vi "Main.vi"(11 "Module Admin":refnum<class "Delacor_lib_QMH_Cloneable Module Admin.lvclass">) -> ()   [LabVIEW 2021, in "Slave.lvlib"]
doc: "This template is based off of the Queued Message Handler design pattern and the Queued Message Handler project template that ships with LabVIEW.\n\nThe main difference is that the queue is private to this module and communication between modules is performed via Broadcast and Request events.\n\nRequest events are wrapped in public API methods and are handled in the Event Handling Loop (EHL) of this VI. Any module can register for Broadcast events sent by this module. The EHL generates messages based on user interface actions.\n\nThe Message Handling Loop (MHL) processes messages generated by the EHL, or by other messages. The messages are string values, so new messages can be added easily to the Message Cases case structure in the MHL. Each message cluster can also provide an optional value for Message Data, which is a variant that can be converted to whatever message-specific data is required.\n_____\nBased on DQMH Project Template 6.1.0.94.\n\n<b>Note:</b> This VI was modified by the <b>Validate DQMH Module</b> tool to add a 'Panel Hidden' status updated broadcast to the Panel Close? event when External Launch = TRUE.\n\n<b>Note:</b> This VI was modified by the <b>Validate DQMH Module</b> tool to add a call to the Error Reported VI at the end of the 'Exit' MHL frame."
uses:
  Slave.lvlib
  <vilib>/Delacor/Delacor QMH/Libraries/Cloneable Module Admin_class/Delacor_lib_QMH_Cloneable Module Admin.lvclass
  C:/Program Files/National Instruments/LabVIEW 2021/vi.lib/Delacor/Delacor QMH/Libraries/Module Admin_class/Delacor_lib_QMH_Module Admin.lvclass
  <vilib>/Delacor/Delacor QMH/Libraries/Cloneable Module Admin_class/Delacor_lib_QMH_Cloneable Module Admin.lvclass/Delacor_lib_QMH_Cloneable Module Admin.ctl
  Module Data--cluster.ctl
  <vilib>/Delacor/Delacor QMH/Libraries/Message Queue_class/Delacor_lib_QMH_Message Queue.lvclass/Delacor_lib_QMH_Message Queue.ctl
  Stop Argument--cluster.ctl
  <vilib>/Delacor/Delacor QMH/Libraries/Module Admin_class/Delacor_lib_QMH_Module Admin.lvclass/Delacor_lib_QMH_Module Admin.ctl
  <vilib>/Utility/miscctls.llb/LVPointTypeDef.ctl
  <vilib>/Delacor/Delacor QMH/Libraries/Message Queue_class/Delacor_lib_QMH_Enqueue Message (Single).vi
  <vilib>/Delacor/Delacor QMH/Libraries/Cloneable Module Admin_class/Delacor_lib_QMH_Get Module ID.vi
  <vilib>/Delacor/Delacor QMH/Libraries/Module Admin_class/Delacor_lib_QMH_Get External Launch.vi
  <vilib>/Utility/error.llb/Error Cluster From Error Code.vi
  <vilib>/ErrorRing/Error Ring.xnode
  <vilib>/Delacor/Delacor QMH/Libraries/Message Queue_class/Delacor_lib_QMH_Message Queue.lvclass
  <vilib>/DQMH Consortium/Lumos API/Libraries/SDV API/SDV API.lvlib
panel:
  out "Title":string
  out "error out":errorcluster
  out "Status":string
  in  "Simulate EHL Error":bool
  in  "Simulate MHL Error":bool
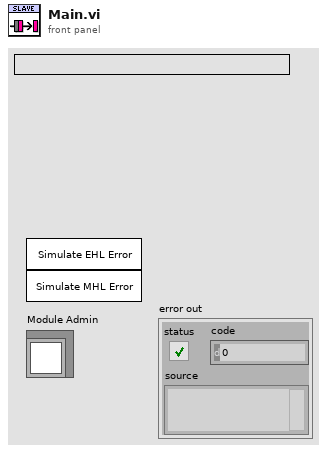
[diagram p1: front panel]
types:
  T1 = typedef "Slave.lvlib/Request Events--cluster.ctl" = cluster{"Stop Module":refnum<user-event>, "Show Panel":refnum<user-event>, "Hide Panel":refnum<user-event>, "Show Diagram":refnum<user-event>, "Get Module Execution Status":refnum<user-event>}
  T2 = typedef "Slave.lvlib/Module Data--cluster.ctl" = cluster{"Status":string}
  T3 = enum32{"invalid lock state", "Not Locked", "Locked (No Password)", "Password-protected"}
  T4 = typedef "Slave.lvlib/Stop Argument--cluster.ctl" = cluster{"Module ID":i32, "Origin":string, "Exit via Stop Module Req?":bool, "Wait for Module to stop?":bool}
  T5 = typedef "LVPointTypeDef.ctl" = cluster{"Horizontal":i16, "Vertical":i16}
  T6 = enum32{"Invalid", "Standard", "Closed", "Hidden", "Minimized", "Maximized"}
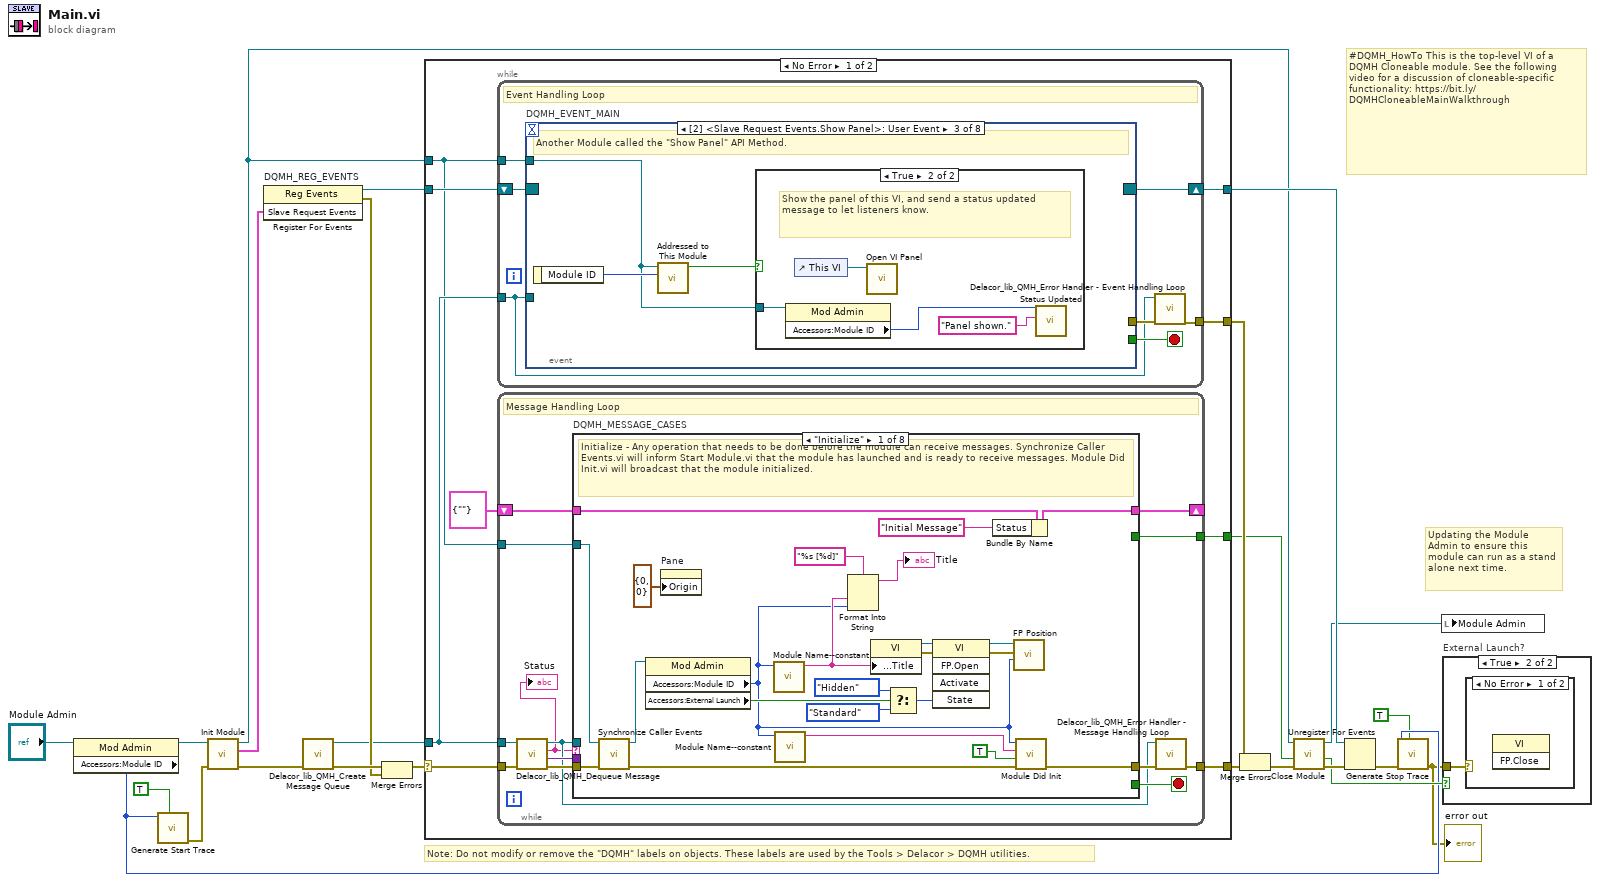
[diagram p0: block diagram]
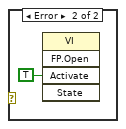
[diagram p3: hidden frame]
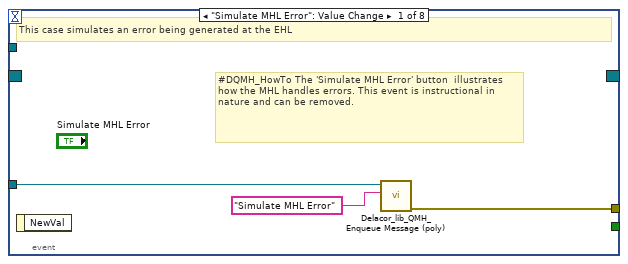
[diagram p4: hidden frame]
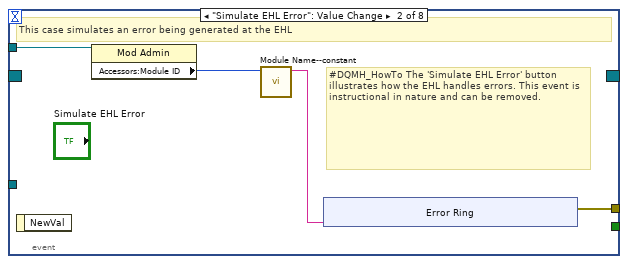
[diagram p5: hidden frame]
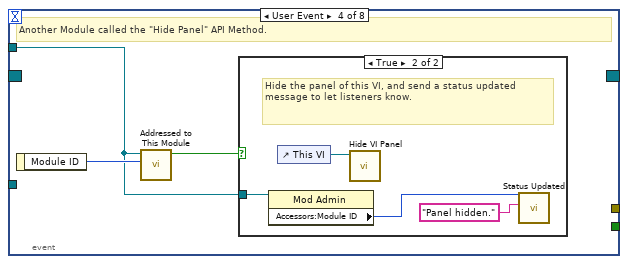
[diagram p7: hidden frame]
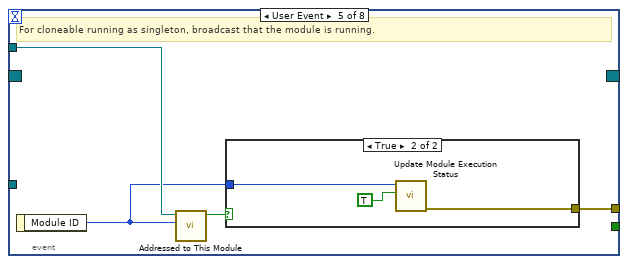
[diagram p9: hidden frame]
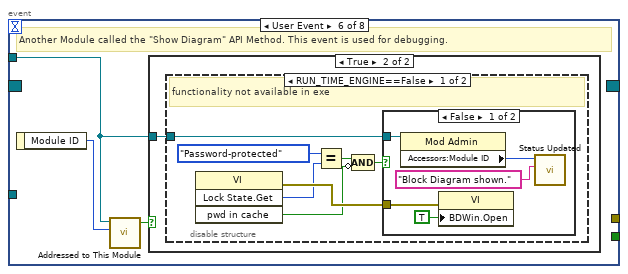
[diagram p11: hidden frame]
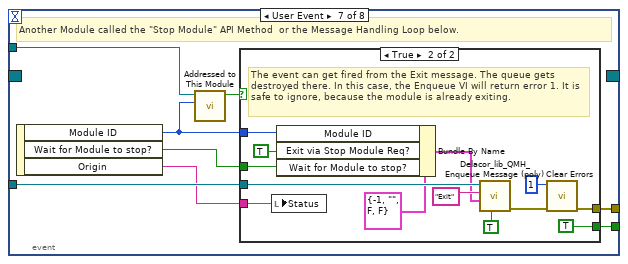
[diagram p15: hidden frame]
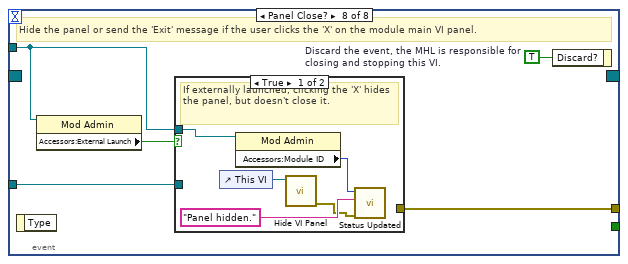
[diagram p17: hidden frame]
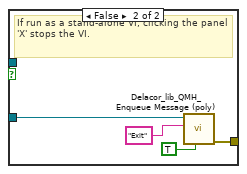
[diagram p18: hidden frame]
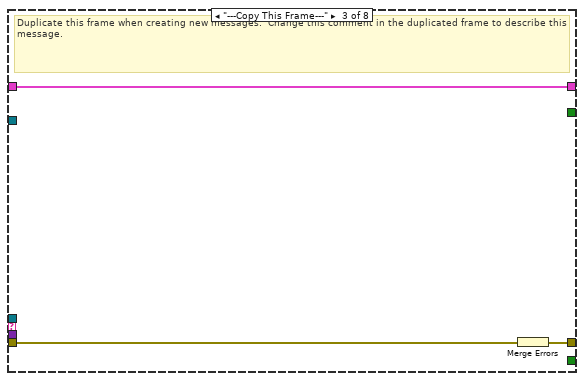
[diagram p20: hidden frame]
diagram:
  # "#DQMH_HowTo This is the top-level VI of a DQMH Cloneable module. See the following video for a discussion of cloneable-specific functionality: https://bit.ly/DQMHCloneableMainWalkthrough"
  # "Note: Do not modify or remove the \"DQMH\" labels on objects. These labels are used by the Tools > Delacor > DQMH utilities."
  # "Updating the Module Admin to ensure this module can run as a stand alone next time."
  n1 = property on="Property Node" class="Mod Admin"(reference="Module Admin") -> (reference out=w6:refnum<class "Delacor_lib_QMH_Cloneable Module Admin.lvclass">, "Accessors:Module ID"=w4:i32)  [unwired: 1 in, 1 out]
  n2 = call <vilib>:"Generate Start Trace.vi"("Reply (F)"=TRUE, "Module ID (0)"=w4) -> ("error out"=w5:errorcluster)  [unwired: 9 in]
  n3 = call "Init Module.vi"("error in"=w5, "Cloneable Module Admin in"=w6) -> ("error out"=w21:errorcluster, "Slave Request Events"=w13:T1, "Cloneable Module Admin out"=w10:refnum<class "Delacor_lib_QMH_Cloneable Module Admin.lvclass">)  [unwired: 7 in]
  n4 = register-events "DQMH_REG_EVENTS"(w13) -> (reference out=w14:refnum<event-registration>, error out=w16:errorcluster)  [unwired: 2 in]
  n5 = call <vilib>:"Delacor_lib_QMH_Create Message Queue.vi"("error in"=w21) -> ("error out"=w18:errorcluster, "Message Queue"=w12:refnum<class "Delacor_lib_QMH_Message Queue.lvclass">)  [unwired: 9 in]
  n6 = Merge Errors(w18, w16) -> (w17:errorcluster)
  n7 = case shown="No Error" w17 {
    selector: w17 -> [w31 w236]
    tunnel: [w33 w235] -> w22
    tunnel: [w30 w243] -> w15
    tunnel: w14 -> [w28 w243]
    tunnel: w12 -> [w27 w234]
    tunnel: [w32 _] -> w23
    tunnel: w10 -> [w26 w239]
    tunnel: [w25 _] -> w8
    frame No Error {
      n8 = while {
        tunnel: w27 -> [w34]
        shift-right: [w37] -> w30
        shift-left: w28 -> [w38]
        tunnel: [w39] -> w32
        tunnel: w26 -> [w35]
        stop <- w36 stop-if-true
        # "Event Handling Loop"
        n9 = event "DQMH_EVENT_MAIN" shown="[2] <Slave Request Events.Show Panel>: User Event" {
          selector: w38 -> [_ _ _ _ _ _ _ _]
          dyn-events: [_ _ _ _ _ _ _ _] -> w37
          timeout: _ -> [_ _ _ _ _ _ _ _]
          tunnel: [_ _ _ _ _ _ w95 _] -> w36
          tunnel: w34 -> [w42 _ _ _ _ _ w98 w115]
          tunnel: [w43 w47 _ _ w72 _ w99 w117] -> w40
          tunnel: w35 -> [_ w46 w55 w62 w70 w76 w97 w113]
          event "Simulate MHL Error": Value Change {
            # "#DQMH_HowTo The 'Simulate MHL Error' button  illustrates how the MHL handles errors. This event is instructional in nature and can be removed."
            # "This case simulates an error being generated at the EHL"
            n10 = event-data() -> ()  [unwired: 1 in, 1 out]
            n11 = call-poly <vilib>:"Delacor_lib_QMH_Enqueue Message (poly).vi"("Message"="Simulate MHL Error", "Message Queue in"=w42) -> ("error out"=w43:errorcluster)  [unwired: 8 in, 1 out]
          }
          event "Simulate EHL Error": Value Change {
            # "#DQMH_HowTo The 'Simulate EHL Error' button  illustrates how the EHL handles errors. This event is instructional in nature and can be removed."
            # "This case simulates an error being generated at the EHL"
            n12 = event-data() -> ()  [unwired: 1 in, 1 out]
            n13 = property on="Property Node" class="Mod Admin"(reference=w46) -> ("Accessors:Module ID"=w45:i32)  [unwired: 1 in, 2 out]
            n14 = call "Module Name--constant.vi"("Module ID"=w45) -> ("Module Name"=w44:string)  [unwired: 10 in]
            n15 = xnode ("Error Ring")("parameter 0"=w44) -> ("error out"=w47:errorcluster)
          }
          event User Event {
            # "Another Module called the \"Show Panel\" API Method."
            n16 = event-data() -> ("Module ID"=w56:i32)  [unwired: 1 in]
            n17 = call "Addressed to This Module.vi"("Module ID from Argument"=w56, "Module Admin"=w55) -> ("Addressed to this instance?"=w57:bool)  [unwired: 8 in, 1 out]
            n18 = case shown="True" w57 {
              tunnel: w55 -> [_ w59]
              frame False {
              }
              frame True {
                # "Show the panel of this VI, and send a status updated message to let listeners know."
                n19 = property on="Property Node" class="Mod Admin"(reference=w59) -> ("Accessors:Module ID"=w58:i32)  [unwired: 1 in, 2 out]
                n20 = control-ref of="This VI"() -> (w61:refnum<vi>)
                n21 = call "Open VI Panel.vi"("VI"=w61) -> ()  [unwired: 10 in, 1 out]
                n22 = call "Status Updated.vi"("Status"="Panel shown." ("format string"), "Module ID"=w58) -> ()  [unwired: 9 in, 1 out]
              }
            }
          }
          event User Event {
            # "Another Module called the \"Hide Panel\" API Method."
            n23 = event-data() -> ("Module ID"=w63:i32)  [unwired: 1 in]
            n24 = call "Addressed to This Module.vi"("Module ID from Argument"=w63, "Module Admin"=w62) -> ("Addressed to this instance?"=w64:bool)  [unwired: 8 in, 1 out]
            n25 = case shown="True" w64 {
              tunnel: w62 -> [_ w66]
              frame False {
              }
              frame True {
                # "Hide the panel of this VI, and send a status updated message to let listeners know."
                n26 = property on="Property Node" class="Mod Admin"(reference=w66) -> ("Accessors:Module ID"=w65:i32)  [unwired: 1 in, 2 out]
                n27 = control-ref of="This VI"() -> (w68:refnum<vi>)
                n28 = call "Hide VI Panel.vi"("VI"=w68) -> ()  [unwired: 10 in, 1 out]
                n29 = call "Status Updated.vi"("Status"="Panel hidden." ("format string"), "Module ID"=w65) -> ()  [unwired: 9 in, 1 out]
              }
            }
          }
          event User Event {
            # "For cloneable running as singleton, broadcast that the module is running."
            n30 = event-data() -> ("Module ID"=w69:i32)  [unwired: 1 in]
            n31 = call "Addressed to This Module.vi"("Module ID from Argument"=w69, "Module Admin"=w70) -> ("Addressed to this instance?"=w71:bool)  [unwired: 8 in, 1 out]
            n32 = case shown="True" w71 {
              tunnel: [_ w75] -> w72
              tunnel: w69 -> [_ w74]
              frame False {
              }
              frame True {
                n33 = call "Update Module Execution Status.vi"("Running?"=TRUE, "Module ID"=w74) -> ("error out"=w75:errorcluster)  [unwired: 9 in]
              }
            }
          }
          event User Event {
            # "Another Module called the \"Show Diagram\" API Method. This event is used for debugging."
            n34 = event-data() -> ("Module ID"=w77:i32)  [unwired: 1 in]
            n35 = call "Addressed to This Module.vi"("Module ID from Argument"=w77, "Module Admin"=w76) -> ("Addressed to this instance?"=w78:bool)  [unwired: 8 in, 1 out]
            n36 = case shown="True" w78 {
              tunnel: w76 -> [_ w79]
              frame False {
              }
              frame True {
                n37 = disable-structure "Conditional Disable Structure" shown="RUN_TIME_ENGINE==False" {
                  disable-tunnel: w79 -> [w80 _]
                  frame condition #0 (active) {
                    # "functionality not available in exe"
                    n38 = invoke on="Invoke Node" class="VI" method="Lock State.Get"() -> (error out=w86:errorcluster, "Get Lock State"=w85:T3, "pwd in cache"=w82:bool)  [unwired: 4 in, 1 out]
                    n39 = Equal?(x=T3."Password-protected", y=w85) -> (x = y?=w83:bool)
                    n40 = Compound Arithmetic op=AND(w83, invert w82) -> (w81:bool)
                    n41 = case shown="False" w81 {
                      tunnel: w86 -> [w91 _]
                      tunnel: w80 -> [w88 _]
                      frame False {
                        n42 = property on="Property Node" class="Mod Admin"(reference=w88) -> ("Accessors:Module ID"=w87:i32)  [unwired: 1 in, 2 out]
                        n43 = property on="Property Node" class="VI"(error in=w91, "BDWin.Open"=TRUE ("Block Diagram Window:Open")) -> ()  [unwired: 1 in, 2 out]
                        n44 = call "Status Updated.vi"("Status"="Block Diagram shown." ("format string"), "Module ID"=w87) -> ()  [unwired: 9 in, 1 out]
                      }
                      frame True {
                        # "Password-protected VI, and the password is not in the cache. Do not show the diagram."
                      }
                    }
                  }
                  frame condition #1 {
                  }
                }
              }
            }
          }
          event User Event {
            # "Another Module called the \"Stop Module\" API Method  or the Message Handling Loop below."
            n45 = event-data() -> ("Module ID"=w93:i32, "Wait for Module to stop?"=w94:bool, "Origin"=w92:string)  [unwired: 1 in]
            n46 = call "Addressed to This Module.vi"("Module ID from Argument"=w93, "Module Admin"=w97) -> ("Addressed to this instance?"=w96:bool)  [unwired: 8 in, 1 out]
            n47 = case shown="True" w96 {
              tunnel: [_ w111] -> w99
              tunnel: w98 -> [_ w107]
              tunnel: [_ TRUE] -> w95
              tunnel: w94 -> [_ w102]
              tunnel: w93 -> [_ w104]
              tunnel: w92 -> [_ w100]
              frame False {
              }
              frame True {
                # "The event can get fired from the Exit message. The queue gets destroyed there. In this case, the Enqueue VI will return error 1. It is safe to ignore, because the module is already exiting."
                n48 = local write "Status"(w100) -> ()
                n49 = Bundle By Name(cluster=T4 {"Module ID"=-1, "Origin"="", "Exit via Stop Module Req?"=FALSE, "Wait for Module to stop?"=FALSE} ("Stop Argument"), "Module ID"=w104, "Exit via Stop Module Req?"=TRUE, "Wait for Module to stop?"=w102) -> (w101:T4)
                n50 = call-poly <vilib>:"Delacor_lib_QMH_Enqueue Message (poly).vi"("Priority Message? (F)"=TRUE, "Message Data"=w101, "Message"="Exit", "Message Queue in"=w107) -> ("error out"=w112:errorcluster)  [unwired: 6 in, 1 out]
                n51 = call <vilib>:"Clear Errors.vi"("error in (no error)"=w112, "specific error code to clear (0: all)"=1) -> ("error out"=w111:errorcluster)  [unwired: 4 in, 1 out]
              }
            }
          }
          event Panel Close? {
            w116 = TRUE  # Discard the event, the MHL is responsible for closing and stopping this VI.
            # "Hide the panel or send the 'Exit' message if the user clicks the 'X' on the module main VI panel."
            n52 = event-data() -> ()  [unwired: 1 in, 1 out]
            n53 = property on="Property Node" class="Mod Admin"(reference=w113) -> ("Accessors:External Launch"=w114:bool)  [unwired: 1 in, 2 out]
            n54 = case shown="True" w114 {
              tunnel: w115 -> [_ w125]
              tunnel: [_ w126] -> w117
              tunnel: w113 -> [w120 _]
              frame True {
                # "If externally launched, clicking the 'X' hides the panel, but doesn't close it."
                n55 = control-ref of="This VI"() -> (w122:refnum<vi>)
                n56 = property class="Mod Admin"(reference=w120) -> ("Accessors:Module ID"=w119:i32)  [unwired: 1 in, 2 out]
                n57 = call "Hide VI Panel.vi"("VI"=w122) -> ("error out"=w118:errorcluster)  [unwired: 10 in]
                n58 = call "Status Updated.vi"("error in (no error)"=w118, "Status"="Panel hidden.", "Module ID"=w119) -> ()  [unwired: 8 in, 1 out]
              }
              frame False {
                # "If run as a stand-alone VI, clicking the panel 'X' stops the VI."
                n59 = call-poly <vilib>:"Delacor_lib_QMH_Enqueue Message (poly).vi"("Priority Message? (F)"=TRUE, "Message"="Exit", "Message Queue in"=w125) -> ("error out"=w126:errorcluster)  [unwired: 7 in, 1 out]
              }
            }
            n60 = event-data ("Event Filter Node")("Discard?"=w116) -> ()  [unwired: 1 in, 1 out]
          }
        }
        n61 = call-dynamic "Delacor_lib_QMH_Error Handler - Event Handling Loop.vi"("error in"=w40, "Message Queue in"=w34) -> ("dup error in"=w39:errorcluster)  [unwired: 8 in, 1 out]
      }
      n62 = while {
        tunnel: w27 -> [w131]
        shift-right: [w134] -> _
        shift-left: T2 {"Status"=""} ("Data Cluster") -> [w135]
        tunnel: w31 -> [w138]
        tunnel: [w136] -> w33
        tunnel: w26 -> [w129]
        tunnel: [w128] -> w25
        stop <- w133 stop-if-true
        # "Message Handling Loop"
        n63 = call-dynamic "Delacor_lib_QMH_Dequeue Message.vi"("error in"=w138, "Message Queue in"=w131) -> ("error out"=w137:errorcluster, "Message Data"=w132:variant, "Message"=w127:string, "Message Queue out"=w130:refnum<class "Delacor_lib_QMH_Message Queue.lvclass">)  [unwired: 6 in]
        "Status" <- w127
        n64 = case "DQMH_MESSAGE_CASES" shown="\"Initialize\"" w127 {
          selector: w127 -> [_ _ _ _ _ _ _ w221]
          tunnel: w130 -> [_ _ _ _ w171 _ w211 _]
          tunnel: w137 -> [w162 w164 w167 w169 w180 w193 w217 w223]
          tunnel: [w160 w164 w166 w169 w176 w192 w214 w224] -> w139
          tunnel: w135 -> [w156 w163 w165 w168 w175 w190 w210 w222]
          tunnel: [w155 w163 w165 w168 w175 w190 w210 w222] -> w134
          tunnel: [_ _ _ _ _ _ w209 _] -> w133
          tunnel: w132 -> [_ _ _ _ w174 _ w207 _]
          tunnel: w129 -> [w151 _ _ _ w173 w188 w203 w219]
          tunnel: [_ _ _ _ _ _ w205 _] -> w128
          frame "Initialize" {
            # "Initialize - Any operation that needs to be done before the module can receive messages. Synchronize Caller Events.vi will inform Start Module.vi that the module has launched and is ready to receive messages. Module Did Init.vi will broadcast that the module initialized."
            n65 = call "Synchronize Caller Events.vi"("error in (no error)"=w162, "Module Admin"=w151) -> ("error out"=w161:errorcluster, "Module Admin out"=w150:refnum<class "Delacor_lib_QMH_Cloneable Module Admin.lvclass">)  [unwired: 8 in]
            n66 = property on="Property Node" class="Mod Admin"(reference=w150) -> ("Accessors:Module ID"=w140:i32, "Accessors:External Launch"=w152:bool)  [unwired: 1 in, 2 out]
            n67 = property on="Pane" class="Pane"("Origin"=T5 {"Horizontal"=0, "Vertical"=0}) -> ()  [unwired: 2 in, 2 out]
            n68 = call "Module Name--constant.vi"("Module ID"=w140) -> ("Module Name"=w145:string)  [unwired: 10 in]
            n69 = call "Module Name--constant.vi"("Module ID"=w140) -> ("Module Name"=w153:string)  [unwired: 10 in]
            n70 = Format Into String(format string="%s [%d]", w145, w140) -> (resulting string=→"Title":string)  [unwired: 2 in, 1 out]
            n71 = property on="Property Node" class="VI"("Front Panel.Title"=w145) -> (reference out=w144:refnum<vi>, error out=w143:errorcluster)  [unwired: 2 in]
            n72 = Select(t=T6."Hidden" ("State"), s=w152, f=T6."Standard" ("State")) -> (s? t:f=w157:T6)
            n73 = invoke on="Invoke Node" class="VI" method="FP.Open"(reference=w144, error in=w143, "State"=w157) -> (reference out=w141:refnum<vi>, error out=w142:errorcluster)  [unwired: 2 in, 3 out]
            n74 = Bundle By Name(cluster=w156, "Status"="Initial Message" ("Initial Message")) -> (w155:T2)
            n75 = call "FP Position.vi"("Module ID"=w140, "error in"=w142, "VI server in"=w141) -> ()  [unwired: 9 in]
            n76 = call "Module Did Init.vi"("error in (no error)"=w161, "Initialized?"=TRUE, "Origin"=w153, "Module ID"=w140) -> ("error out"=w160:errorcluster)  [unwired: 7 in]
          }
          frame "---Module Specific---" {
            # "Separator -- The following cases handle messages specific to this Module."
          }
          frame "---Copy This Frame---" {
            # "Duplicate this frame when creating new messages.  Change this comment in the duplicated frame to describe this message."
            n77 = Merge Errors(w167) -> (w166:errorcluster)
          }
          frame "---Exit and Error Handling---" {
            # "Separator - the following cases handle errors and exit messages."
          }
          frame "Error" {
            # "#CodeRecommended - If you ever change the name of this \"Error\" message, you'll need to update the name in the Check Loop Error.vi as well."
            # "#CodeRecommended - If the module is running in standalone mode (External Launch = FALSE), this code will pop up an error dialog and call the 'Exit' message if an error occurs. Add more fine-grained error handling here."
            # "Error - Check the error message data and respond accordingly. This message is sent by the \"Error Handler\" VIs at the end of each loop in this application."
            n78 = property on="Property Node" class="Mod Admin"(reference=w173) -> ("Accessors:External Launch"=w172:bool, "Accessors:Module ID"=w170:i32)  [unwired: 1 in, 2 out]
            n79 = Variant To Data(error in=w180, type=errorcluster {"status"=FALSE, "code"=0, "source"=""} ("error constant"), Variant=w174) -> (data=w181:errorcluster, error out=w178:errorcluster)
            n80 = call "Error Reported.vi"("Error"=w181, "Module ID"=w170) -> ()  [unwired: 9 in, 1 out]
            n81 = case shown="False" w172 {
              tunnel: [w186 _] -> w177
              tunnel: w171 -> [w184 _]
              tunnel: w181 -> [w185 _]
              frame False {
                # "If the module is running standalone, then pop up an error dialog and call the \"Exit\" message."
                n82 = call <vilib>:"Simple Error Handler.vi"("error in (no error)"=w185) -> ()  [unwired: 4 in, 5 out]
                n83 = call-poly <vilib>:"Delacor_lib_QMH_Enqueue Message (poly).vi"("Priority Message? (F)"=TRUE, "Message"="Exit", "Message Queue in"=w184) -> ("error out"=w186:errorcluster)  [unwired: 7 in, 1 out]
              }
              frame True {
                # "If the module was launched externally, calling the Error Reported broadcast VI is the only action performed by the \"Error\" message. The module's caller can then process the error appropriately."
              }
            }
            n84 = Merge Errors(w178, w177) -> (w176:errorcluster)
            n85 = local write "error out"(w176) -> ()
          }
          frame "Simulate MHL Error" {
            # "#DQMH_HowTo The 'Simulate MHL Error' button  illustrates how the MHL handles errors. This event is instructional in nature and can be removed."
            # "Simulate an error occurring at the MHL"
            n86 = property on="Property Node" class="Mod Admin"(reference=w188) -> ("Accessors:Module ID"=w189:i32)  [unwired: 1 in, 2 out]
            n87 = call "Module Name--constant.vi"("Module ID"=w189) -> ("Module Name"=w187:string)  [unwired: 10 in]
            n88 = xnode ("Error Ring")("parameter 0"=w187) -> ("error out"=w191:errorcluster)
            n89 = Merge Errors(w193, w191) -> (w192:errorcluster)
          }
          frame "Exit" {
            w208 = 91  # 91: not all Exit messages will have an argument
            w209 = TRUE  # Stop the VI
            # "Release the message queue reference"
            # "#CodeNeeded - Add any required cleanup code here."
            # "Exit - Exit the application."
            n90 = Variant To Data(error in=w217, type=T4 {"Module ID"=-1, "Origin"="", "Exit via Stop Module Req?"=FALSE, "Wait for Module to stop?"=FALSE} ("Stop Argument"), Variant=w207) -> (data=w204:T4, error out=w212:errorcluster)
            n91 = call <vilib>:"Clear Errors.vi"("error in (no error)"=w212, "specific error code to clear (0: all)"=w208) -> ("error out"=w216:errorcluster)  [unwired: 4 in, 1 out]
            n92 = control-ref of="This VI"() -> (w202:refnum<vi>)
            n93 = call-dynamic "Delacor_lib_QMH_Release Message Queue.vi"("error in"=w216, "Message Queue"=w211) -> ("error out"=w215:errorcluster)  [unwired: 9 in]
            n94 = call "Handle Exit.vi"("Stop Argument"=w204, "Module Admin in"=w203, "VI reference"=w202) -> ("error out"=w213:errorcluster, "Wait for Stop?"=w205:bool)  [unwired: 7 in]
            n95 = property class="Mod Admin"(reference=w203) -> ("Accessors:Module ID"=w201:i32)  [unwired: 1 in, 2 out]
            n96 = Merge Errors(w215, w213) -> (w214:errorcluster)
            n97 = call "Error Reported.vi"("Error"=w214, "Module ID"=w201) -> ()  [unwired: 9 in, 1 out]
          }
          frame Default {
            # "'Default' case only runs if there is a message that isn't defined in any of the other cases.  Output a programming error."
            n98 = property on="Property Node" class="Mod Admin"(reference=w219) -> ("Accessors:Module ID"=w218:i32)  [unwired: 1 in, 2 out]
            n99 = call "Module Name--constant.vi"("Module ID"=w218) -> ("Module Name"=w220:string)  [unwired: 10 in]
            n100 = xnode ("Error Ring")("parameter 0"=w221, "parameter 1"=w220) -> ("error out"=w225:errorcluster)
            n101 = Merge Errors(w223, w225) -> (w224:errorcluster)
          }
        }
        n102 = call-dynamic "Delacor_lib_QMH_Error Handler - Message Handling Loop.vi"("error in"=w139, "Message Queue in"=w130) -> ("dup error in"=w136:errorcluster)  [unwired: 8 in, 1 out]
      }
    }
    frame Error {
      n103 = call "Synchronize Caller Events.vi"("Module Admin"=w239) -> ("Module Admin out"=w238:refnum<class "Delacor_lib_QMH_Cloneable Module Admin.lvclass">)  [unwired: 9 in, 1 out]
      n104 = property on="Property Node" class="Mod Admin"(reference=w238) -> ("Accessors:Module ID"=w237:i32)  [unwired: 1 in, 2 out]
      n105 = call-dynamic "Delacor_lib_QMH_Release Message Queue.vi"("error in"=w236, "Message Queue"=w234) -> ("error out"=w235:errorcluster)  [unwired: 9 in]
      n106 = call "Module Name--constant.vi"("Module ID"=w237) -> ("Module Name"=w242:string)  [unwired: 10 in]
      n107 = Format Into String(format string="An error occurred during initialization. %s is no longer running.", w242) -> (resulting string=w240:string)  [unwired: 2 in, 1 out]
      n108 = call "Error Reported.vi"("Additional Information"=w240, "Error"=w235, "Module ID"=w237) -> ()  [unwired: 8 in, 1 out]
    }
  }
  n109 = Merge Errors(w23, w22) -> (w24:errorcluster)
  n110 = call "Close Module.vi"("error in"=w24, "Wait for stop?"=w8, "Module Admin in"=w10) -> ("error out"=w20:errorcluster, "External Launch"=w7:bool, "Module Admin out"=w9:refnum<class "Delacor_lib_QMH_Cloneable Module Admin.lvclass">)  [unwired: 6 in]
  n111 = Unregister For Events(event registration refnum=w15, error in=w20) -> (error out=w19:errorcluster)
  n112 = call <vilib>:"Generate Stop Trace.vi"("Reply (F)"=TRUE, "error in (no error)"=w19, "Module ID (0)"=w4) -> ("error out"=w2:errorcluster)  [unwired: 8 in]
  "error out" <- w2
  n113 = local write "Module Admin"(w9) -> ()
  n114 = case "External Launch?" shown="True" w7 {
    tunnel: w2 -> [_ w244]
    frame False {
    }
    frame True {
      n115 = case shown="No Error" w244 {
        frame No Error {
          n116 = invoke on="Invoke Node" class="VI" method="FP.Close"() -> ()  [unwired: 3 in, 3 out]
        }
        frame Error {
          n117 = invoke on="Invoke Node" class="VI" method="FP.Open"("Activate"=TRUE ("Activate?")) -> ()  [unwired: 4 in, 5 out]
        }
      }
    }
  }
